vi "Read Single Device.vi"(6 "Index":i32, 7 "Section":string, 8 "error in (no error)":errorcluster, 9 "Key Names":string[](array[string]), 10 "Platforms":refnum<class "PlatformManager.lvclass">, 11 "refnum":T1) -> (0 "error out":errorcluster, 1 "Remaining Key Names":string[](array[string]), 3 "refnum out":T1, 5 "Device":refnum<class "Device.lvclass">)   [LabVIEW 2020, in "PicoG-App.lvlib" / "picoG.lvclass"]
uses:
  picoG.lvclass
  <vilib>/Utility/config.llb/Config Data RefNum.ctl
  Device/Device.lvclass
  Builds/picoG/ppl/PicoG-Core.lvlibp/PicoG-Processor/PicoG-Core/PlatformManager/PlatformManager.lvclass
  Device/Device Key.ctl
  Builds/picoG/ppl/PicoG-Core.lvlibp/PicoG-Processor/PicoG-Core/Resource/Resource.lvclass
  Builds/picoG/ppl/PicoG-Core.lvlibp/PicoG-Processor/PicoG-Core/Resource/Config Item.ctl
  <vilib>/Utility/config.llb/Read Key (String).vi
  <vilib>/Utility/config.llb/NI_LVConfig.lvlib
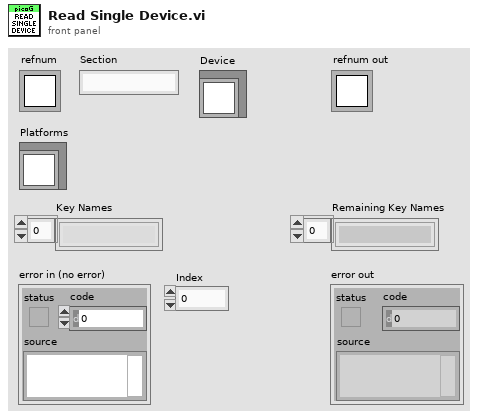
[diagram p1: front panel]
types:
  T1 = typedef "NI_LVConfig.lvlib/Config Data RefNum.ctl" = refnum<k1>
  T2 = typedef "PicoG-App.lvlib/Device.lvclass/Device Key.ctl" = cluster{"Platform":string, "Board":string, "ID":string}
  T3 = typedef "PicoG-Core.lvlibp/Resource.lvclass/Config Item.ctl" = cluster{"Key":string, "Value":string}
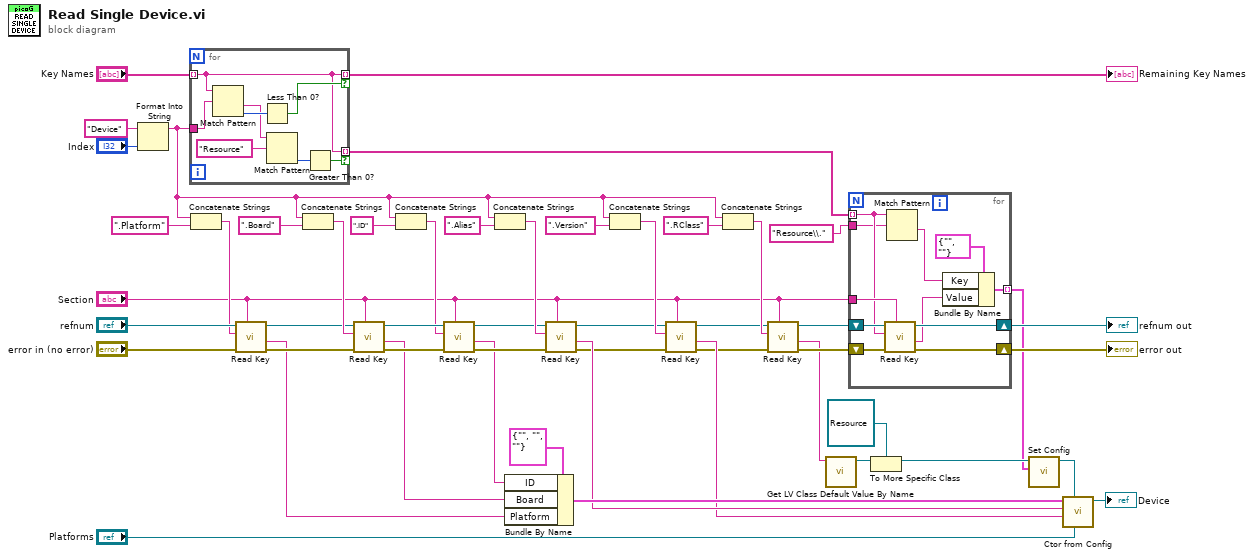
[diagram p0: block diagram]
diagram:
  n1 = Format Into String(initial string="Device", "Index") -> (resulting string=w17:string)  [unwired: 2 in, 1 out]
  n2 = for {
    tunnel: "Key Names" -> [w53] mode=indexing
    tunnel: w17 -> [w59]
    tunnel: [w53] -> w49 mode=indexing if=w57
    tunnel: [w53] -> w20 mode=indexing if=w52
    n3 = Match Pattern(string=w53, regular expression=w59) -> (after substring=w56:string, offset past match=w58:i32)  [unwired: 1 in, 2 out]
    n4 = Less Than 0?(x=w58) -> (x < 0?=w57:bool)
    n5 = Match Pattern(string=w56, regular expression="Resource") -> (offset past match=w54:i32)  [unwired: 1 in, 3 out]
    n6 = Greater Than 0?(x=w54) -> (x > 0?=w52:bool)
  }
  "Remaining Key Names" <- w49
  n7 = Concatenate Strings(w17, ".Platform" ("string")) -> (w41:string)
  n8 = call-poly <vilib>:"Read Key.vi"("section"="Section", "error in (no error)"="error in (no error)", "key"=w41, "refnum"="refnum") -> ("error out"=w38:errorcluster, "value"=w29:string, "refnum out"=w39:T1)  [unwired: 4 in, 1 out]
  n9 = Concatenate Strings(w17, ".Board" ("string")) -> (w40:string)
  n10 = call-poly <vilib>:"Read Key.vi"("section"="Section", "error in (no error)"=w38, "key"=w40, "refnum"=w39) -> ("error out"=w36:errorcluster, "value"=w28:string, "refnum out"=w37:T1)  [unwired: 4 in, 1 out]
  n11 = Concatenate Strings(w17, ".ID" ("string")) -> (w35:string)
  n12 = call-poly <vilib>:"Read Key.vi"("section"="Section", "error in (no error)"=w36, "key"=w35, "refnum"=w37) -> ("error out"=w32:errorcluster, "value"=w27:string, "refnum out"=w33:T1)  [unwired: 4 in, 1 out]
  n13 = Concatenate Strings(w17, ".Alias" ("string")) -> (w34:string)
  n14 = Bundle By Name(cluster=T2 {"Platform"="", "Board"="", "ID"=""} ("Device Key"), "ID"=w27, "Board"=w28, "Platform"=w29) -> (w30:T2)
  n15 = call-poly <vilib>:"Read Key.vi"("section"="Section", "error in (no error)"=w32, "key"=w34, "refnum"=w33) -> ("error out"=w21:errorcluster, "value"=w26:string, "refnum out"=w22:T1)  [unwired: 4 in, 1 out]
  n16 = Concatenate Strings(w17, ".Version" ("string")) -> (w23:string)
  n17 = call-poly <vilib>:"Read Key.vi"("section"="Section", "error in (no error)"=w21, "key"=w23, "refnum"=w22) -> ("error out"=w14:errorcluster, "value"=w25:string, "refnum out"=w15:T1)  [unwired: 4 in, 1 out]
  n18 = Concatenate Strings(w17, ".RClass" ("string")) -> (w16:string)
  n19 = call-poly <vilib>:"Read Key.vi"("section"="Section", "error in (no error)"=w14, "key"=w16, "refnum"=w15) -> ("error out"=w12:errorcluster, "value"=w10:string, "refnum out"=w11:T1)  [unwired: 4 in, 1 out]
  n20 = call <vilib>:"Get LV Class Default Value By Name.vi"("class name"=w10) -> ("object"=w9:refnum<class>)  [unwired: 9 in, 1 out]
  n21 = for {
    shift-right: [w66] -> w5
    shift-left: w12 -> [w70]
    shift-right: [w67] -> w6
    shift-left: w11 -> [w69]
    tunnel: "Section" -> [w68]
    tunnel: w20 -> [w65] mode=indexing
    tunnel: "Resource\\." ("regular expression") -> [w64]
    tunnel: [w60] -> w4 mode=indexing
    n22 = call-poly <vilib>:"Read Key.vi"("section"=w68, "error in (no error)"=w70, "key"=w65, "refnum"=w69) -> ("error out"=w66:errorcluster, "value"=w62:string, "refnum out"=w67:T1)  [unwired: 4 in, 1 out]
    n23 = Match Pattern(string=w65, regular expression=w64) -> (after substring=w61:string)  [unwired: 1 in, 3 out]
    n24 = Bundle By Name(cluster=T3 {"Key"="", "Value"=""} ("Config Item"), "Key"=w61, "Value"=w62) -> (w60:T3)
  }
  "error out" <- w5
  "refnum out" <- w6
  n25 = To More Specific Class(target class=refnum<class "Resource.lvclass"> refnum ("Resource"), reference=w9) -> (specific class reference=w7:refnum<class "Resource.lvclass">)  [unwired: 1 in, 1 out]
  n26 = call "Set Config.vi"("Config"=w4, "DeployResource in"=w7) -> ("DeployResource out"=w3:refnum<class "Resource.lvclass">)  [unwired: 8 in, 1 out]
  n27 = call "Ctor from Config.vi"("Platforms"="Platforms", "Resource"=w3, "Version"=w25, "Alias"=w26, "Device Key"=w30) -> ("Device out"=→"Device":refnum<class "Device.lvclass">)  [unwired: 5 in, 1 out]
